vi "Evaluate Part 1.vi"() -> ()   [LabVIEW 2020]
uses:
  Proto/NetAn.lvclass
panel:
  out "size(s)":i32
  in  "Input":string="kh-tc\nqp-kh\nde-cg\nka-co\nyn-aq\nqp-ub\ncg-tb\nvc-aq\ntb-ka\nwh-tc\nyn-cg\nkh-ub\nta-co\nde-co\ntc-td\ntb-wq\nwh-td\nta-ka\ntd-qp\naq-cg\nwq-ub\nub-vc\nde-ta\nwq-aq\nwq-vc\nwh-yn\nka-de\nkh-ta\nco-tc\nwh-qp\ntb-vc\ntd-yn"
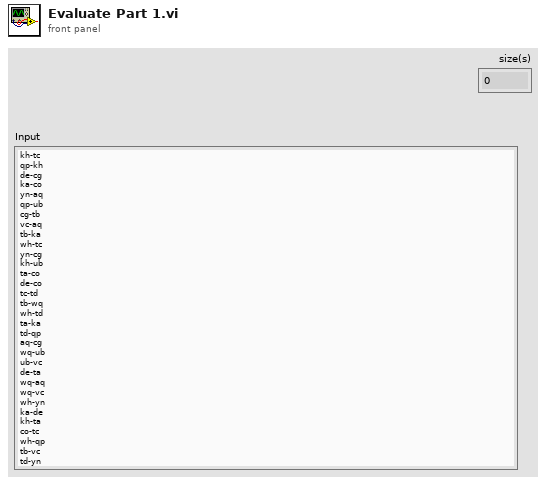
[diagram p1: front panel]
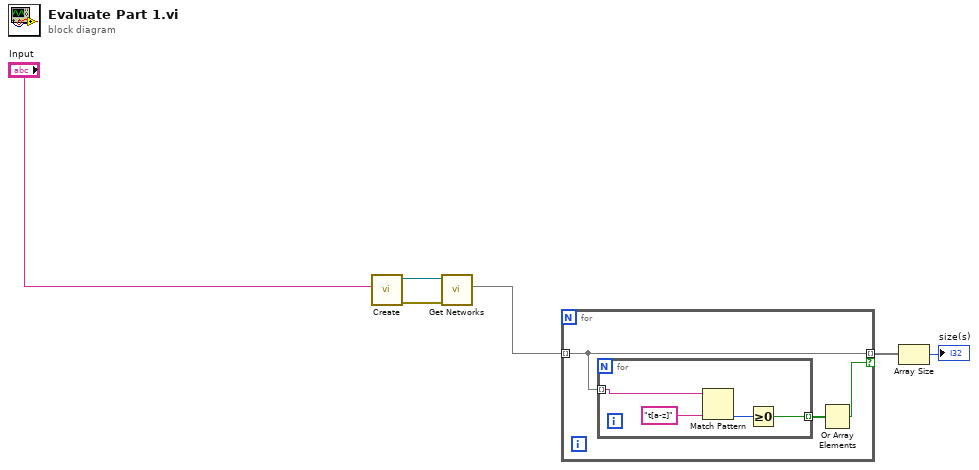
[diagram p0: block diagram]
diagram:
  n1 = call "Create.vi"("Input"="Input") -> ("error out"=w4:errorcluster, "Proto"=w5:refnum<class "NetAn.lvclass">)  [unwired: 9 in]
  n2 = call "Get Networks.vi"("error in (no error)"=w4, "Proto in"=w5) -> ("set"=w3:set{set{string}})  [unwired: 7 in, 2 out]
  n3 = for {
    tunnel: w3 -> [w8] mode=indexing
    tunnel: [w8] -> w2 mode=indexing if=w7
    n4 = for {
      tunnel: w8 -> [w13] mode=indexing
      tunnel: [w10] -> w9 mode=indexing
      n5 = Match Pattern(string=w13, regular expression="t[a-z]") -> (offset past match=w11:i32)  [unwired: 1 in, 3 out]
      n6 = Greater Or Equal To 0?(x=w11) -> (x >= 0?=w10:bool)
    }
    n7 = Or Array Elements(Boolean array=w9) -> (logical OR=w7:bool)
  }
  n8 = Array Size(array=w2) -> (size(s)=→"size(s)":i32)
